vi "datatype2string.vi"(11 "datatype":T1(ring)) -> (3 "Ring Text.Text":string)   [LabVIEW 2014]
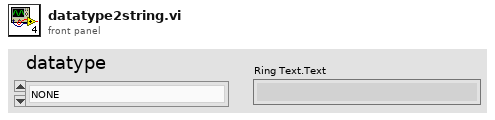
[diagram p1: front panel]
types:
  T1 = enum16{"NONE", "BINARY", "UNSIGNED_CHAR", "SIGNED_SHORT", "SIGNED_INT", "FLOAT", "COMPLEX", "DOUBLE", "RGB", "ALL"}
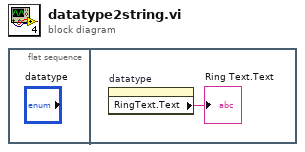
[diagram p0: block diagram]
diagram:
  n1 = flat-sequence {
    frame #0 {
    }
    frame #1 {
      n2 = property on="datatype" class="Enum (strict)"() -> ("RingText.Text"=→"Ring Text.Text":string)  [unwired: 2 in, 2 out]
    }
  }
